vi "Dashboard Main.vi"() -> ()   [LabVIEW 2017]
uses:
  <vilib>/Rock Robotics/WPI/DriverStation/WPI_DriverStationAllianceInfo.ctl
  <vilib>/Utility/miscctls.llb/LVRowAndColumnTypeDef.ctl
  <vilib>/event_ctls.llb/eventvkey.ctl
  <vilib>/Rock Robotics/Network Tables/NT Read Numeric Array.vi
  <vilib>/Rock Robotics/WPI/Dashboard/WPI_DashboardLogging Global.vi
  <vilib>/Rock Robotics/Network Tables/NT Write Numeric Array.vi
  <vilib>/Rock Robotics/Network Tables/NT Write Boolean.vi
  <vilib>/Rock Robotics/Network Tables/NT Read Boolean.vi
panel:
  out "NT Connection":bool=TRUE
  in  "Camera Settings Right":T1={"Frame Rate"=15, "Compression"=30, "Size"=1, "DB Camera Config"=FALSE} {"Frame Rate" scale=1.0..30.0; "Compression" scale=100.0..-1.0; "Size" items=["640x480", "320x240", "160x120"]}
  in  "Camera Name Right":string(combo)="No Camera Selection"
  out "Camera Info":cluster{"Mbps LED":bool, "Mbps":dbl, "fps":dbl}={"Mbps LED"=FALSE, "Mbps"=0.17652911574406902, "fps"=9.930486593843098} {"fps" format="%#.1g"; "Mbps" format="%#.1g"}
  in  "Camera Settings":T1={"Frame Rate"=10, "Compression"=66, "Size"=2, "DB Camera Config"=FALSE} {"Frame Rate" scale=1.0..30.0; "Compression" scale=100.0..-1.0; "Size" items=["640x480", "320x240", "160x120"]}
  in  "TCP":refnum<k5>
  in  "Rec Mode":enum32{"Stop", "Record", "Playback"}(radio)
  out "Robot IP":string="10.17.12.2"
  out "Image Message":string="Timeout in Camera Communications"
  in  "Dashboard Tab":T2(tab)
  in  "Reset":bool
  out "HasCube":bool
  out "Mode":T3(ring)
  out "Gyro":dbl(knob)=-172.57 scale=-180.0..180.0
  out "Elevator":dbl(slide)=5.727272727272727 scale=-10.0..80.0
  out "LeftEncoder":dbl=817.74403425
  out "RightEncoder":dbl=362.091195
  out "Bottom":bool
  out "Top":bool
  out "Camera Image Right":T4(plugin-control)
  in  "DB/String 9":string
  in  "DB/String 8":string
  in  "DB/String 7":string
  in  "DB/String 6":string
  in  "DB/String 5":string
  in  "DB/String 4":string
  in  "DB/String 3":string
  in  "DB/String 2":string
  in  "DB/String 1":string
  in  "DB/String 0":string
  in  "DB/Slider 0":dbl(slide) scale=0.0..5.0
  in  "DB/Slider 1":dbl(slide) scale=0.0..5.0
  in  "DB/Slider 2":dbl(slide) scale=0.0..5.0
  in  "DB/Slider 3":dbl(slide) scale=0.0..5.0
  out "DB/LED 3":bool
  out "DB/LED 2":bool
  out "DB/LED 1":bool
  out "DB/LED 0":bool
  in  "DB/Button 3":bool
  in  "DB/Button 2":bool
  in  "DB/Button 1":bool
  in  "DB/Button 0":bool caption="New Name"
  in  "RR Delay":dbl
  in  "LR Delay":dbl
  in  "LL Delay":dbl
  in  "RRAction2":dbl
  in  "LRAction2":dbl
  in  "LLAction2":dbl
  in  "RRAction1":dbl
  in  "LRAction1":dbl
  in  "LLAction1":dbl
  in  "NotPurePursuit":bool
  in  "Battery Number":string
  out "?":bool=TRUE
  out "Opponent Right Switch":bool
  out "Center Left Scale":bool=TRUE
  out "Center Right Scale":bool
  out "Our Left Team Switch":bool=TRUE
  out "Our Right Team Switch":bool
  in  "Position":u32=3
  in  "RLAction1":dbl
  in  "RLAction2":dbl
  in  "RL Delay":dbl
  in  "Test Slider":dbl(slide) scale=0.0..100.0 scale format="%#_3g"
  in  "On/Off":bool caption="Solenoid"
  in  "Test Name":u16(ring) items=["Select the test to run..."]
  in  "Test Tree":string(tree)
  in  "Motor":cluster{"Value":dbl, "Enable":bool} {"Value" scale=-1.0..1.0 scale format="%#_3g"}
  out "Progress":T5 {"Test Progress" scale=0.0..100.0}
  in  "Rev/Fwd":cluster{"Forward":bool, "Reverse":bool}
  in  "Test Ring":u16(ring) items=["Monochrome", "Color"]
  out "Cmd Status":string
  in  "Execute Command":bool
  in  "Command Params":string[][](table)
  in  "Command Selection":i32(listbox)
  in  "CheckList":i32(listbox)
  out "Tree":string(tree)
  out "Camera Image":T4(plugin-control)
  in  "Camera Name":string(combo)="Camera"
  # "Don't use this row"
  # "HW"
  # "HW"
  # "Switch/Scale Positions"
  # "1Cube"
  # "2Cube"
  # "Delay"
  # "Left"
  # "Left"
  # "Right"
  # "Left"
  # "Left"
  # "Right"
  # "Right"
  # "Right"
  # "Action Key:\n0 = Do Nothing\n1 = Go Switch\n2 = Go Scale"
  # "1"
  # "2"
  # "3"
  # "4"
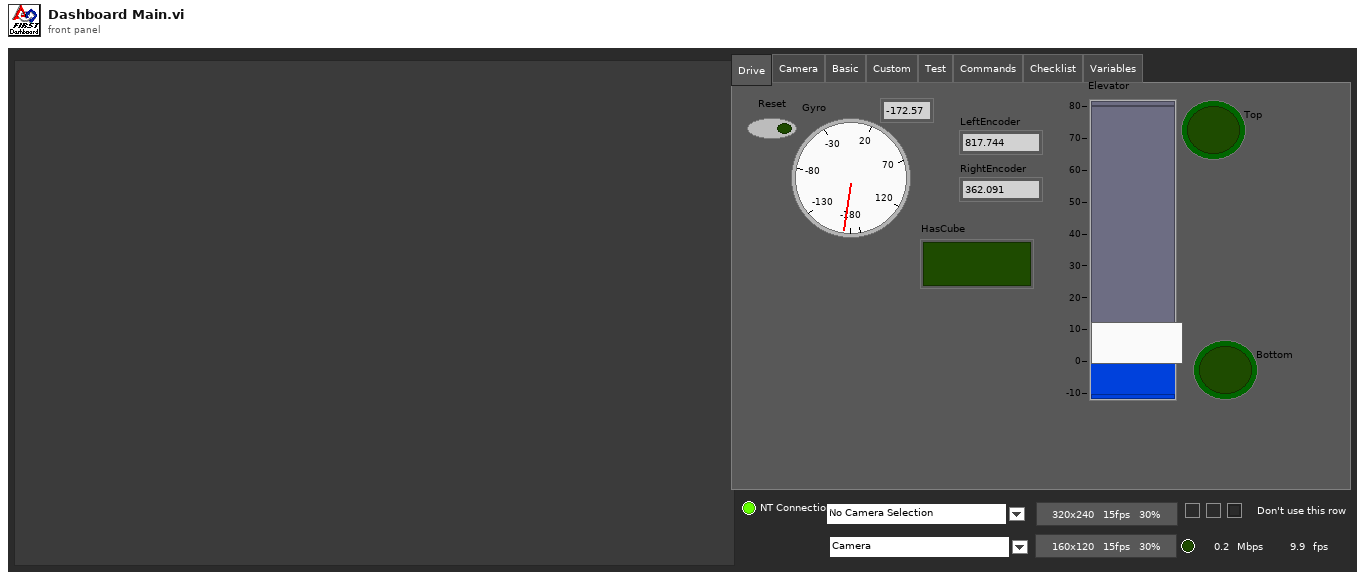
[diagram p1: front panel]
types:
  T1 = cluster{"Frame Rate":i32, "Compression":i32, "Size":u16, "DB Camera Config":bool}
  T2 = enum32{"Drive", "Camera", "Basic", "Custom", "Test", "Commands", "Checklist", "Variables"}
  T3 = enum8{"Tele-Op Disabled", "Tele-Op Enabled", "Auto Disabled", "Auto Enabled", "Test Disabled", "Test Enabled", "Disconnected", "No Code", "E-Stop"}
  T4 = typedef "IMAQ Image.ctl" = refnum<image>
  T5 = cluster{"Test Progress":u8, "Test Progress Text":string}
  T6 = cluster{"Save Path":path, "Interval (s)":dbl, "Keep":i32}
  T7 = typedef "Image Type" = u32
  T8 = cluster{"IDs":cluster{"RPC field ID":u16, "Unique ID":u16}, "String":string}
  T9 = cluster{"Camera Image":refnum<vi>, "Dashboard Tab":refnum<vi>, "Rec Mode":refnum<vi>, "Test Slider":refnum<vi>, "On/Off ":refnum<vi>, "Test Ring":refnum<vi>, "Rev/Fwd":refnum<vi>, "Test Name":refnum<vi>, "Motor":refnum<vi>, "Progress":refnum<vi>, "CheckList":refnum<vi>, "Tree":refnum<vi>, "Test Tree":refnum<vi>, "Command Params":refnum<vi>, "Command Selection":refnum<vi>, "Execute Command":refnum<vi>, "Cmd Status":refnum<vi>, "Camera Settings":refnum<vi>, "Camera Name":refnum<vi>, "Camera Info":refnum<vi>, "Camera Settings Right":refnum<vi>, "Camera Name Right":refnum<vi>, "Camera Image Right":refnum<vi>}
  T10 = cluster{"Error Strings":string, "Disable Counts":cluster{u16, u16}, "Rail Faults":cluster{u16, u16, u16}, "Robot IP":string, "DB Mode":u8, "Event Info":cluster{"Name":string, "Type":u8, "Number":u16, "Replay":u8}}
  T11 = cluster{"Storage":cluster{"Disk Free":u64, "RAM Block":u32, "RAM free":u32}, "CPU Utilization":cluster{"CPU % ISR":sgl, "CPU % Time Crit":sgl, "CPU % Timed Str":sgl, "CPU % High":sgl, "CPU % Above":sgl, "CPU % Normal":sgl, "CPU % Low":sgl}, "CAN":cluster{"% Bus Utilization":sgl, "Bus Off Cnt":u32, "TX_FIFO Full Cnt":u32, "Receive Error Cnt":u8, "Transmit Error Cnt":u8}, "HID":cluster{"HID Outputs":u32, "Rumble Low":u16, "Rumble High":u16}[]}
  T12 = cluster{"Status bits":cluster{"Test Mode":bool, "Autonomous":bool, "Enabled":bool, "Code Start":bool, "Brownout":bool, "Reserved 2":bool, "Reserved 3":bool, "E-Stop":bool}, "Code Trace":cluster{"Disabled":bool, "TeleOp":bool, "Auto":bool, "Test":bool}, "Controller Type":enum16{"unknown", "cRIO", "roboRio"}, "Code?":enum16{"unknown", "noCode", "code"}, "Battery V":dbl}
  T13 = cluster{"Control Bits":cluster{"TestMode":bool, "Autonomous":bool, "Enabled":bool, "FMS Present":bool, bool, bool, bool, "E-Stop":bool}, "Team Station ":u8, "Countdown":sgl, "Joystick Values":cluster{"Axes":dbl[], "Buttons":bool[], "POVs":i16[]}[]}
  T14 = cluster{"Axes":dbl[], "Buttons":bool[], "POVs":i16[]}[]
  T15 = cluster{"Axes":dbl[], "Buttons":bool[], "POVs":i16[]}
  T16 = cluster{"Camera Name":string, string, "Saved DB Images Info":cluster{"Save Path":path, "Interval (s)":dbl, "Keep":i32}}
  T17 = cluster{"Camera Name Right":string, string, "Saved DB Images Info":cluster{"Save Path":path, "Interval (s)":dbl, "Keep":i32}}
  T18 = cluster{"Operation":enum16{"Update", "Clear"}, "Color Box":u32}[]
  T19 = typedef "eventvkey.ctl" = enum16{"ASCII", "Enter", "Return", "Shift", "Ctrl", "Alt", "Cmd", "Opt", "Caps", "NumLock", "Clear", "Break", "Up", "Down", "Left", "Right", "Insert", "Delete", "Home", "End", "PageUp", "PageDown", "Escape", "Help", "Pause", "ScrollLock", "F1", "F2", "F3", "F4", "F5", "F6", "F7", "F8", "F9", "F10", "F11", "F12", "F13", "F14", "F15", "F16", "F17", "F18", "F19", "F20", "F21", "F22", "F23", "F24", "Play", "VolumeUp", "VolumeDown", "Mute", "Two Byte Char"}
  T20 = cluster{"Image Size":bool, "Image Type":bool, "Pixel Value":bool, "ROI Information":bool, "Zoom Factor":bool}
  T21 = cluster{"Operation":enum16{"Update", "Clear"}, "Color Box":u32}
  T22 = typedef "LVRowAndColumnTypeDef.ctl" = cluster{"Row":i32, "Column":i32}
  T23 = cluster{"Shift":bool, "Ctrl":bool, "Alt":bool, "Cmd":bool, "Opt":bool}
  T24 = typedef "WPI_DriverStationAllianceInfo.ctl" = enum16{"Red", "Blue", "Invalid"}
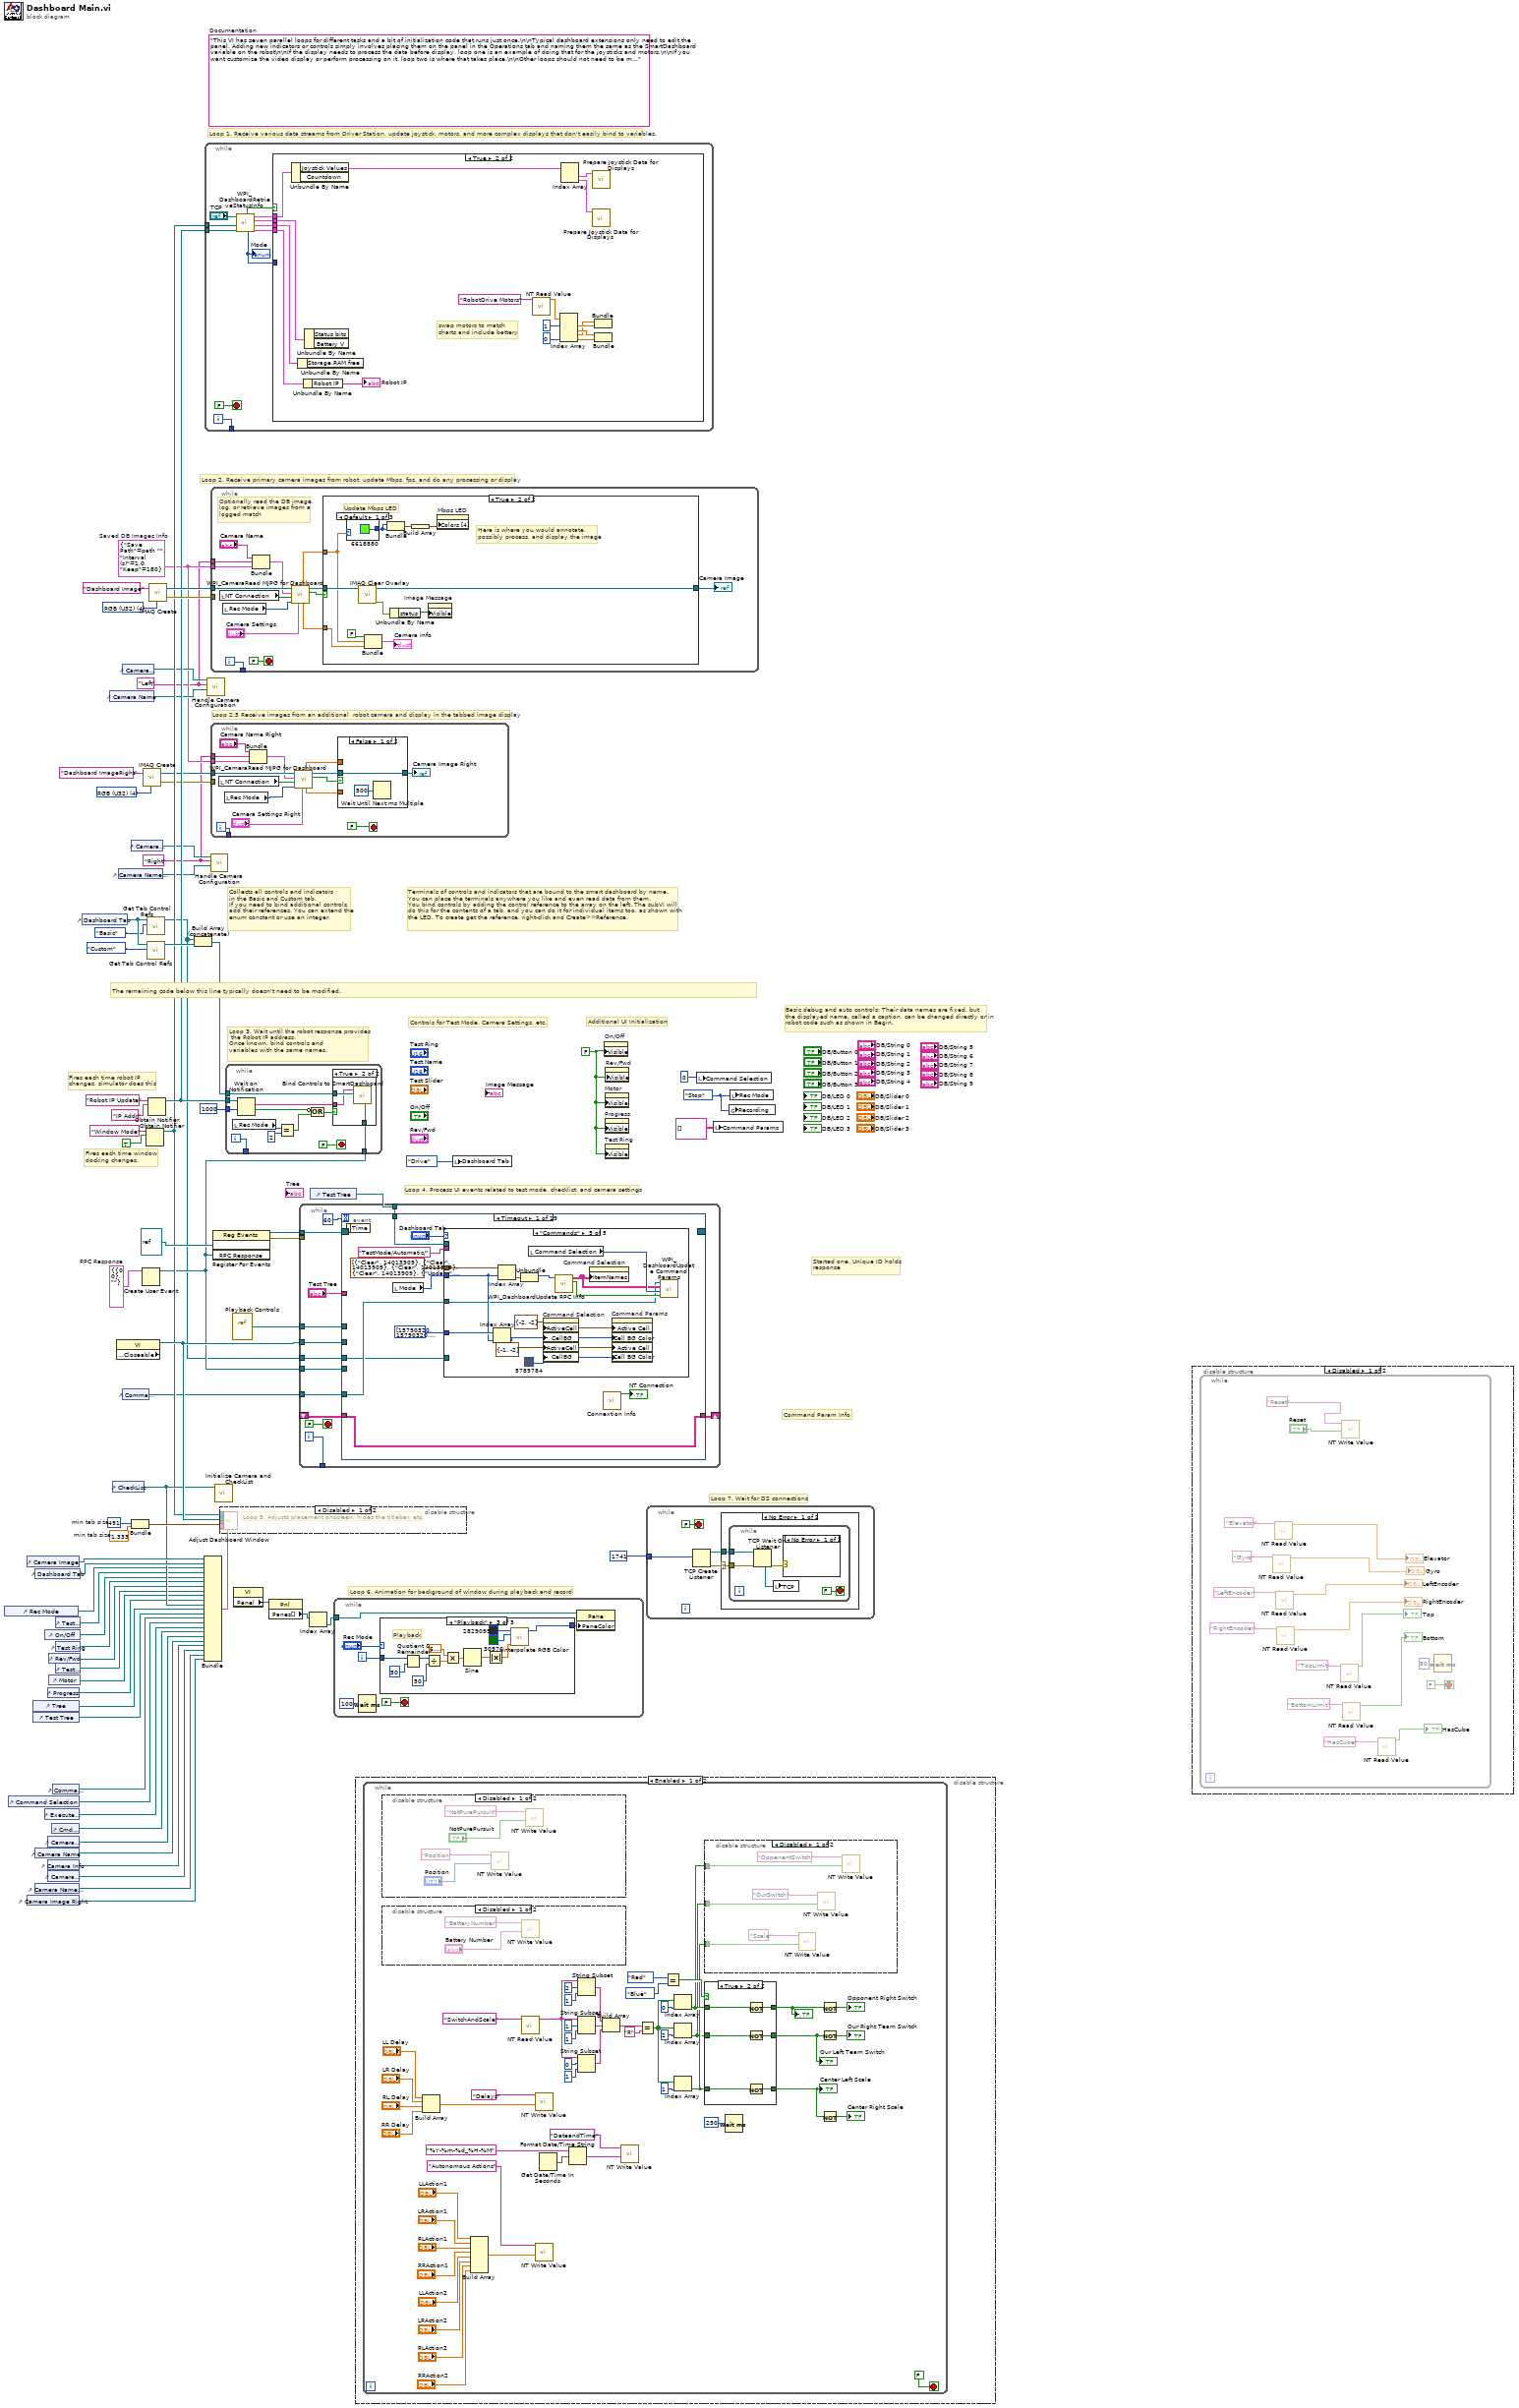
[diagram p0: block diagram]
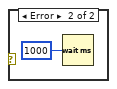
[diagram p10: hidden frame]
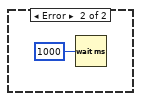
[diagram p11: hidden frame]
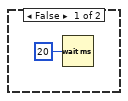
[diagram p12: hidden frame]
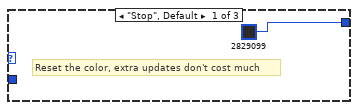
[diagram p13: hidden frame]
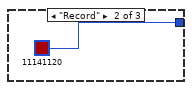
[diagram p14: hidden frame]
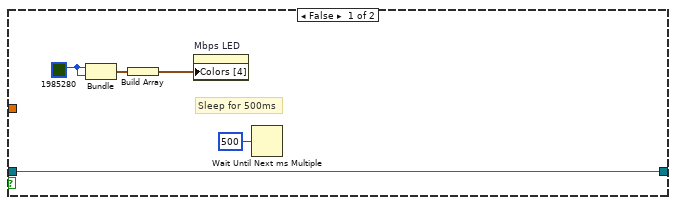
[diagram p16: hidden frame]
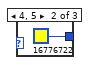
[diagram p17: hidden frame]
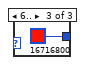
[diagram p18: hidden frame]
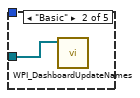
[diagram p20: hidden frame]
diagram:
  w4 = T6 {"Save Path"=path "", "Interval (s)"=1.0, "Keep"=180}  # Saved DB Images Info
  w3 = "Right"
  w2 = "Left"
  w14 = T7 4 items=["Grayscale (U8)", "Grayscale (I16)", "Grayscale (SGL)", "Complex (CSG)", "RGB (U32)", "HSL (U32)", "RGB (U64)"] ("Image Type")
  w28 = T8 {"IDs"={"RPC field ID"=0, "Unique ID"=0}, "String"=""}  # RPC Response
  w49 = 491  # min tab size
  w48 = 1.333  # min tab size
  w56 = enum32{"Stop", "Record", "Playback"}."Stop" ("Rec Mode")
  w34 = FALSE ("Visible")
  (unwired) "This VI has seven parallel loops for different tasks and a bit of initialization code that runs just once.\n\nTypical dashboard extensions only need to edit the panel. Adding new indicators or controls simply involves placing them on the panel in the Operations tab and naming them the same as the SmartDashboard variable on the robot\n\nIf the display needs to process the data before display, loop one is an example of doing that for the joysticks and motors.\n\nIf you want customize the video display or perform processing on it, loop two is where that takes place.\n\nOther loops should not need to be modified. They are pretty standard, and document the task they perform."  # Documentation
  w73 = T7 4 items=["Grayscale (U8)", "Grayscale (I16)", "Grayscale (SGL)", "Complex (CSG)", "RGB (U32)", "HSL (U32)", "RGB (U64)"] ("Image Type")
  # "Loop 2.5 Receive images from an additional  robot camera and display in the tabbed image display"
  # "Command Param Info"
  # "Started one, Unique ID holds\nresponse"
  # "Loop 7. Wait for DS connections"
  # "Basic debug and auto controls: Their data names are fixed, but\nthe displayed name, called a caption, can be changed directly or in\nrobot code such as shown in Begin."
  # "Controls for Test Mode, Camera Settings, etc."
  # "Additional UI Initialization"
  # "Loop 6. Animation for background of window during playback and record"
  # "Fires each time robot IP\nchanges, simulator does this"
  # "Fires each time window\ndocking changes."
  # "Collects all controls and indicators\nin the Basic and Custom tab.\nIf you need to bind additional controls,\nadd their references. You can extend the\nenum constant or use an integer."
  # "The remaining code below this line typically doesn't need to be modified."
  # "Loop 4. Process UI events related to test mode, checklist, and camera settings"
  # "Terminals of controls and indicators that are bound to the smart dashboard by name.\nYou can place the terminals anywhere you like and even read data from them.\nYou bind controls by adding the control reference to the array on the left. The subVI will\ndo this for the contents of a tab, and you can do it for individual items too, as shown with\nthe LED. To create get the reference, right-click and Create>>Reference."
  # "Loop 3. Wait until the robot response provides\n the Robot IP address.\nOnce known, bind controls and\nvariables with the same names."
  # "Loop 1. Receive various data streams from Driver Station, update joystick, motors, and more complex displays that don't easily bind to variables."
  # "Loop 2. Receive primary camera images from robot, update Mbps, fps, and do any processing or display"
  n1 = control-ref of="Rec Mode"() -> (w40:refnum<vi>)
  n2 = control-ref of="Command Selection"() -> (w27:refnum<vi>)
  n3 = control-ref of="Camera Image Right"() -> (w7:refnum<vi>)
  n4 = control-ref of="Camera Image"() -> (w51:refnum<vi>)
  n5 = control-ref of="Tree"() -> (w44:refnum<vi>)
  n6 = control-ref of="Test Tree"() -> (w43:refnum<vi>)
  n7 = control-ref of="Dashboard Tab"() -> (w50:refnum<vi>)
  n8 = control-ref of="Camera Name"() -> (w18:refnum<vi>)
  n9 = control-ref of="Camera Name Right"() -> (w8:refnum<vi>)
  n10 = control-ref of="Execute Command"() -> (w29:refnum<vi>)
  n11 = control-ref of="On/Off"() -> (w38:refnum<vi>)
  n12 = control-ref of="Progress"() -> (w35:refnum<vi>)
  n13 = control-ref of="Camera Settings"() -> (w19:refnum<vi>)
  n14 = control-ref of="Camera Info"() -> (w17:refnum<vi>)
  n15 = control-ref of="Camera Settings Right"() -> (w9:refnum<vi>)
  n16 = control-ref of="Rev/Fwd"() -> (w36:refnum<vi>)
  n17 = control-ref of="Motor"() -> (w41:refnum<vi>)
  n18 = control-ref of="Cmd Status"() -> (w23:refnum<vi>)
  n19 = control-ref of="Command Params"() -> (w30:refnum<vi>)
  n20 = control-ref of="Test Slider"() -> (w39:refnum<vi>)
  n21 = control-ref of="Test Ring"() -> (w37:refnum<vi>)
  n22 = control-ref of="Test Name"() -> (w42:refnum<vi>)
  n23 = control-ref of="Dashboard Tab"() -> (w54:refnum<vi>)
  n24 = control-ref of="Camera Name"() -> (w20:refnum<vi>)
  n25 = control-ref of="CheckList"() -> (w45:refnum<vi>)
  n26 = property class="VI" props=["Front Panel.Closeable"]() -> (reference out=w55:refnum<vi>)  [unwired: 2 in, 2 out]
  n27 = control-ref of="Camera Name Right"() -> (w10:refnum<vi>)
  n28 = control-ref of="Camera Settings"() -> (w21:refnum<vi>)
  n29 = control-ref of="Command Params"() -> (w22:refnum<vi>)
  n30 = control-ref of="Camera Settings Right"() -> (w11:refnum<vi>)
  n31 = Bundle("min tab size"=w49, "min tab size"=w48) -> (w47:cluster{"min tab size":i32, "min tab size":dbl})  [unwired: 1 in]
  n32 = Create User Event(user event datatype=w28) -> (user event=w24:refnum<user-event>)  [unwired: 1 in, 1 out]
  n33 = call "IMAQ Create"("Image Name"="Dashboard ImageRight", "Image Type"=w14) -> ("New Image"=w13:T4, "error out"=w12:errorcluster)  [unwired: 2 in, 1 out]
  n34 = Obtain Notifier(name (unnamed)="Window Mode", notification data type=TRUE) -> (notifier out=w32:refnum<notifier>)  [unwired: 2 in, 2 out]
  n35 = call <vilib>:"Get Tab Control Refs.vi"("Page Index"=T2."Basic" ("Dashboard Tab"), "TabControl in"=w54) -> ("ControlsOnPage"=w16:refnum<vi>[])  [unwired: 9 in]
  n36 = call <vilib>:"Get Tab Control Refs.vi"("Page Index"=T2."Custom" ("Dashboard Tab"), "TabControl in"=w54) -> ("ControlsOnPage"=w53:refnum<vi>[])  [unwired: 9 in]
  n37 = Obtain Notifier(name (unnamed)="Robot IP Update", notification data type="IP Addr" ("name (unnamed)")) -> (notifier out=w33:refnum<notifier>)  [unwired: 2 in, 2 out]
  n38 = call "IMAQ Create"("Image Name"="Dashboard Image", "Image Type"=w73) -> ("New Image"=w71:T4, "error out"=w70:errorcluster)  [unwired: 2 in, 1 out]
  n39 = Build Array (concatenate)(w16, w53) -> (w52:refnum<vi>[])
  n40 = Bundle("Camera Image"=w51, "Dashboard Tab"=w50, "Rec Mode"=w40, "Test Slider"=w39, "On/Off"=w38, "Test Ring"=w37, "Rev/Fwd"=w36, "Test Name"=w42, "Motor"=w41, "Progress"=w35, "CheckList"=w45, "Tree"=w44, "Test Tree"=w43, "Command Params"=w30, "Command Selection"=w27, "Execute Command"=w29, "Cmd Status"=w23, "Camera Settings"=w19, "Camera Name"=w18, "Camera Info"=w17, "Camera Settings Right"=w9, "Camera Name Right"=w8, "Camera Image Right"=w7) -> (w46:T9)  [unwired: 1 in]
  n41 = while {
    tunnel: [w83] -> _
    tunnel: w33 -> [w77]
    tunnel: w32 -> [w74]
    i -> [w83]
    stop <- FALSE stop-if-true
    n42 = call <vilib>:"WPI_DashboardRetrieveStatusInfo.vi"("Binding Refnum"=w77, "Window Mode Notifier"=w74, "TCP Cnx"="TCP") -> ("Power and Errors"=w78:T10, "Robot Metrics"=w81:T11, "Status Info"=w82:T12, "Control Info"=w79:T13, "Robot Mode"=w76:T3, "Process?"=w80:bool)  [unwired: 3 in]
    "Mode" <- w76
    n43 = case shown="True" w80 {
      tunnel: w82 -> [_ w101]
      tunnel: w81 -> [_ w100]
      tunnel: w79 -> [_ w99]
      tunnel: w78 -> [_ w98]
      tunnel: w76 -> [_ _]
      frame False {
        n44 = Wait (ms)(milliseconds to wait=u32 20) -> ()  [unwired: 1 out]
      }
      frame True {
        # "swap motors to match\ncharts and include battery"
        n45 = Unbundle By Name(w99) -> ("Joystick Values"=w91:T14)  [unwired: 1 out]
        n46 = Unbundle By Name(w100) -> ()  [unwired: 1 out]
        n47 = Unbundle By Name(w98) -> ("Robot IP"=→"Robot IP":string)
        n48 = Unbundle By Name(w101) -> ()  [unwired: 2 out]
        n49 = call-poly <vilib>:"NT Read Value.vi"("Name"="RobotDrive Motors") -> ("Numeric Array"=w87:dbl[])  [unwired: 9 in, 1 out]
        n50 = Index Array(array=w87, index #1=1, index #4=0) -> (element #1=w93:dbl, element #2=w94:dbl, element #3=w92:dbl, element #4=w97:dbl)  [unwired: 2 in]
        n51 = Index Array(array=w91) -> (element #1=w90:T15, element #2=w89:T15)  [unwired: 2 in]
        n52 = call "Prepare Joystick Data for Displays.vi"("Joystick Values"=w89) -> ()  [unwired: 8 in, 3 out]
        n53 = call "Prepare Joystick Data for Displays.vi"("Joystick Values"=w90) -> ()  [unwired: 8 in, 3 out]
        n54 = Bundle("Numeric"=w92, "Numeric"=w93) -> ()  [unwired: 1 in, 1 out]
        n55 = Bundle("Numeric"=w94, "Numeric"=w97) -> ()  [unwired: 1 in, 1 out]
      }
    }
  }
  n56 = call "Handle Camera Configuration.vi"("CameraNameRef"=w20, "Display Name"=w2, "ClusterRef"=w21) -> ()  [unwired: 9 in]
  n57 = while {
    tunnel: w71 -> [w114]
    tunnel: w70 -> [_]
    tunnel: [w115] -> _
    tunnel: w4 -> [w105]
    tunnel: w2 -> [w102]
    i -> [w115]
    stop <- FALSE stop-if-true
    # "Optionally read the DB image,\nlog, or retrieve images from a\nlogged match"
    n58 = local read "NT Connection"() -> (w106:bool)
    n59 = local read "Rec Mode"() -> (w110:enum32{"Stop", "Record", "Playback"})
    n60 = Bundle("Camera Name"="Camera Name", w102, "Saved DB Images Info"=w105) -> (w104:T16)  [unwired: 1 in]
    n61 = call <vilib>:"WPI_CameraRead MJPG for Dashboard.vi"("Camera Settings"="Camera Settings", "Rec Mode"=w110, "NT Connection"=w106, "Capture Info"=w104, "Refnum in"=w114) -> ("Active"=w112:bool, "Refnum out"=w113:T4, "FPS"=w111:dbl, "Bandwidth (Mbps)"=w109:dbl)  [unwired: 3 in]
    n62 = case shown="True" w112 {
      tunnel: w113 -> [w117 w128]
      tunnel: w109 -> [_ w125]
      tunnel: w111 -> [_ w126]
      tunnel: [w117 w122] -> w107
      frame False {
        w119 = u32 1985280 ("Color Box")
        # "Sleep for 500ms"
        n63 = Bundle("Color Box"=w119, "Color Box"=w119) -> (w120:cluster{"Color Box":u32, "Color Box":u32})  [unwired: 1 out]
        n64 = Build Array(w120) -> (w118:cluster{"Color Box":u32, "Color Box":u32}[])
        n65 = property on="Mbps LED" class="Bool (strict)"("Colors [4]"=w118) -> ()  [unwired: 2 in, 2 out]
        n66 = Wait Until Next ms Multiple(millisecond multiple=u32 500) -> ()  [unwired: 1 out]
      }
      frame True {
        # "Here is where you would annotate,\npossibly process, and display the image"
        # "Update Mbps LED"
        n67 = case shown="Default" w125 {
          tunnel: [u32 6618880 ("Color Box") u32 16776722 ("Color Box") u32 16716800 ("Color Box")] -> w129
          frame Default {
          }
          frame 4, 5 {
          }
          frame 6.. {
          }
        }
        n68 = call "IMAQ Clear Overlay"("Image"=w128) -> ("error out"=w131:errorcluster, "Image Out"=w122:T4)  [unwired: 2 in, 7 out]
        n69 = Bundle(FALSE, "Bandwidth (Mbps)"=w125, "FPS"=w126) -> (→"Camera Info":cluster{bool, "Bandwidth (Mbps)":dbl, "FPS":dbl})  [unwired: 1 in]
        n70 = Bundle("Color Box"=w129, "Color Box"=w129) -> (w130:cluster{"Color Box":u32, "Color Box":u32})  [unwired: 1 out]
        n71 = Unbundle By Name(w131) -> ("status"=w132:bool)
        n72 = Build Array(w130) -> (w127:cluster{"Color Box":u32, "Color Box":u32}[])
        n73 = property on="Image Message" class="Str"("Visible"=w132) -> ()  [unwired: 2 in, 2 out]
        n74 = property on="Mbps LED" class="Bool (strict)"("Colors [4]"=w127) -> ()  [unwired: 2 in, 2 out]
      }
    }
    "Camera Image" <- w107
  }
  n75 = while {
    tunnel: w13 -> [w150]
    tunnel: w12 -> [_]
    tunnel: [w145] -> _
    tunnel: w4 -> [w139]
    tunnel: w3 -> [w136]
    i -> [w145]
    stop <- FALSE stop-if-true
    n76 = local read "NT Connection"() -> (w140:bool)
    n77 = local read "Rec Mode"() -> (w149:enum32{"Stop", "Record", "Playback"})
    n78 = Bundle("Camera Name Right"="Camera Name Right", w136, "Saved DB Images Info"=w139) -> (w138:T17)  [unwired: 1 in]
    n79 = call <vilib>:"WPI_CameraRead MJPG for Dashboard.vi"("Camera Settings"="Camera Settings Right", "Rec Mode"=w149, "NT Connection"=w140, "Capture Info"=w138, "Refnum in"=w150) -> ("Active"=w144:bool, "Refnum out"=w147:T4, "FPS"=w142:dbl, "Bandwidth (Mbps)"=w143:dbl)  [unwired: 3 in]
    n80 = case shown="False" w144 {
      tunnel: w147 -> [w151 w153]
      tunnel: w143 -> [_ _]
      tunnel: w142 -> [_ _]
      tunnel: [w151 w153] -> w141
      frame False {
        n81 = Wait Until Next ms Multiple(millisecond multiple=u32 500) -> ()  [unwired: 1 out]
      }
      frame True {
      }
    }
    "Camera Image Right" <- w141
  }
  n82 = call "Handle Camera Configuration.vi"("CameraNameRef"=w10, "Display Name"=w3, "ClusterRef"=w11) -> ()  [unwired: 9 in]
  n83 = register-events(refnum<vi> refnum, w24) -> (reference out=w60:refnum<event-registration>, error out=w59:errorcluster)  [unwired: 2 in]
  n84 = call "Initialize Camera and CheckList.vi"("ListBox in"=w45) -> ()  [unwired: 11 in]
  n85 = disable-structure shown="Disabled" {
    disable-tunnel: w55 -> [w157 _]
    disable-tunnel: w47 -> [w156 _]
    disable-tunnel: w46 -> [w155 _]
    disable-tunnel: w32 -> [w154 _]
    frame Disabled {
      # "Loop 5. Adjusts placement onscreen, hides the titlebar, etc."
      n86 = call "Adjust Dashboard Window.vi"("Sizing Refnums"=w155, "Size Constraints"=w156, "VI"=w157, "WIn Mode"=w154) -> ()  [unwired: 8 in]
    }
    frame Enabled {
    }
  }
  n87 = while {
    tunnel: w52 -> [w169]
    tunnel: w33 -> [w167]
    tunnel: [w165] -> _
    tunnel: u32 1000 ("milliseconds to wait") -> [w164]
    tunnel: w24 -> [w158]
    i -> [w165]
    stop <- FALSE stop-if-true
    n88 = local read "Rec Mode"() -> (w160:enum32{"Stop", "Record", "Playback"})
    n89 = Wait on Notification(notifier=w167, timeout in ms (-1)=w164) -> (notification=w166:string, timed out?=w162:bool)  [unwired: 2 in, 2 out]
    n90 = Equal?(x=w160, y=u16 2 ("Rec Mode")) -> (x = y?=w161:bool)
    n91 = Compound Arithmetic op=OR(invert w162, w161) -> (w163:bool)
    n92 = case shown="True" w163 {
      tunnel: w169 -> [_ w172]
      tunnel: w166 -> [_ w171]
      tunnel: w158 -> [_ w170]
      frame False {
      }
      frame True {
        n93 = call <vilib>:"Bind Controls to SmartDashboard.vi"("RPC ref"=w170, "Bound Control Refs"=w172, "Server IP Address"=w171) -> ()  [unwired: 9 in]
      }
    }
  }
  n94 = vi-ref "Playback Controls.vi"() -> (w61:refnum<vi>)
  n95 = property class="VI"() -> ("Panel"=w63:refnum<vi>)  [unwired: 2 in, 2 out]
  n96 = property class="Pnl"(reference=w63) -> ("Panes[]"=w64:refnum<vi>[])  [unwired: 1 in, 2 out]
  n97 = Index Array(array=w64) -> (element=w62:refnum<vi>)  [unwired: 1 in]
  n98 = control-ref of="Test Tree"() -> (w65:refnum<vi>)
  n99 = while {
    tunnel: [w182] -> _
    tunnel: w65 -> [w181]
    tunnel: w61 -> [w180]
    tunnel: w60 -> [w179]
    tunnel: w59 -> [_]
    tunnel: w55 -> [w178]
    tunnel: w24 -> [w177]
    tunnel: w22 -> [w176]
    shift-right: [w175] -> _
    shift-left: _ -> [w174]
    tunnel: w16 -> [w173]
    i -> [w182]
    stop <- FALSE stop-if-true
    n100 = event shown="[0] Timeout" {
      selector: w179 -> [_ _ _ _ _ _ _ _ _ _ _ _ _ _ _ _ _ _ _]
      dyn-events: [_ _ _ _ _ _ _ _ _ _ _ _ _ _ w436 _ _ _ _] -> _
      timeout: u32 60 ("milliseconds to wait") -> [_ _ _ _ _ _ _ _ _ _ _ _ _ _ _ _ _ _ _]
      tunnel: w181 -> [w194 _ _ _ _ _ _ _ _ _ _ _ _ _ _ _ _ _ _]
      tunnel: "Test Tree" -> [_ _ _ _ _ _ _ _ _ w403 w411 w413 w417 w425 _ _ _ _ _]
      tunnel: w180 -> [_ _ _ _ _ _ _ _ _ _ _ _ _ _ w438 _ w456 _ _]
      tunnel: w178 -> [_ _ _ _ _ _ _ _ _ _ _ _ _ _ w434 _ _ _ _]
      tunnel: w177 -> [_ _ _ _ _ _ _ _ _ _ _ _ _ _ w432 _ _ _ _]
      tunnel: w176 -> [w189 _ _ _ w354 _ _ _ _ _ _ _ _ _ _ _ _ _ _]
      tunnel: [w188 w237 w339 w344 w352 w361 w371 w378 w390 w402 w409 w412 w416 w424 w431 w451 w453 w457 w470] -> w175
      tunnel: w174 -> [w188 w237 w339 w344 w352 _ _ w378 w390 w402 w409 w412 w416 w424 w431 w451 w453 w457 w470]
      tunnel: w173 -> [w186 _ _ _ _ _ _ _ _ _ _ _ _ _ _ _ _ _ _]
      event Timeout {
        n101 = event-data() -> ()  [unwired: 1 in, 1 out]
        n102 = local read "Mode"() -> (w191:T3)
        n103 = case shown="\"Commands\"" "Dashboard Tab" {
          tunnel: w194 -> [_ _ w210 _ _]
          tunnel: "TestMode/Automatic/" ("Name Pattern") -> [_ _ w209 _ _]
          tunnel: T18 [{"Operation"=enum."Clear", "Color Box"=14013909}, {"Operation"=enum."Clear", "Color Box"=14013909}, {"Operation"=enum."Clear", "Color Box"=14013909}, {"Operation"=enum."Clear", "Color Box"=14013909}, {"Operation"=enum."Update", "Color Box"=14013909}, {"Operation"=enum."Update", "Color Box"=16777215}, {"Operation"=enum."Clear", "Color Box"=14013909}, {"Operation"=enum."Clear", "Color Box"=14013909}, {"Operation"=enum."Clear", "Color Box"=14013909}] -> [_ _ w202 _ w230]
          tunnel: w191 -> [_ _ w201 _ w229]
          tunnel: u32[] [15790320, 15790320, 15790320, 15790320, 16777215, 16777215, 15790320, 15790320, 15790320] -> [_ _ _ _ w235]
          tunnel: w189 -> [_ _ _ _ w223]
          tunnel: w186 -> [_ w196 _ _ _]
          frame "Custom", Default {
          }
          frame "Basic" {
            n104 = call <vilib>:"WPI_DashboardUpdateNames.vi"("Controls on Tab"=w196) -> ()  [unwired: 11 in]
          }
          frame "Test" {
            w208 = -2 ("Active Item:Row Number")
            n105 = Index Array(array=w202, index=w201) -> (element=w203:T21)
            n106 = Unbundle(w203) -> ("Operation"=w204:enum16{"Update", "Clear"}, "Color Box"=w205:u32)
            n107 = call <vilib>:"NT Read String.vi"("Name"="TestMode/TestName") -> ("String"=w199:string)  [unwired: 9 in, 1 out]
            n108 = call <vilib>:"NT Read and Format Entries as Tree.vi"("Operation"=w204, "Name Pattern"=w209, "Tree Refnum"=w210) -> ()  [unwired: 7 in, 2 out]
            n109 = case shown="\"\"" w199 {
              tunnel: "TestMode/TestProgress" ("Name") -> [w212 _]
              tunnel: "TestMode/TestProgressText" ("Name") -> [w211 _]
              frame Default {
                n110 = call <vilib>:"NT Read Number.vi"("Name"=w212) -> ("Numeric"=w213:dbl)  [unwired: 9 in, 1 out]
                n111 = call <vilib>:"NT Read String.vi"("Name"=w211) -> ("String"=w214:string)  [unwired: 9 in, 1 out]
                n112 = Bundle("Numeric"=w213, "String"=w214) -> (→"Progress":cluster{"Numeric":dbl, "String":string})  [unwired: 1 in]
              }
              frame "" {
                n113 = property on="Progress" class="Clust (strict)"("Visible"=FALSE) -> ()  [unwired: 2 in, 2 out]
                n114 = local write "Test Name"(u16 0) -> ()
              }
            }
            n115 = property on="Test Tree" class="Tree (strict)"("Active Item Row Number"=w208, "ActiveColNum"=w208, "CellBG"=w205, "Active Item Row Number"=-1 ("Active Item:Row Number"), "CellBG"=u32 5789784 ("Color Box")) -> ()  [unwired: 2 in, 2 out]
          }
          frame "Variables" {
            w220 = string[] ["CameraPublisher", "Usage", "DB"]  # Items to initially close
            n116 = First Call?() -> (First Call?: T/F=w221:bool)
            n117 = control-ref of="Tree"() -> (w222:refnum<vi>)
            n118 = Select(t=w220, s=w221, f=string[] []) -> (s? t:f=w218:string[])
            n119 = call <vilib>:"NT Read and Format Entries as Tree.vi"("Tags to  Close"=w218, "Tree Refnum"=w222) -> ()  [unwired: 8 in, 2 out]
          }
          frame "Commands" {
            w231 = u32 5789784 ("Color Box")
            w232 = T22 {"Row"=-1, "Column"=-2} ("Active Cell:Active Cell")
            w234 = T22 {"Row"=-2, "Column"=-2} ("Active Cell:Active Cell")
            n120 = Index Array(array=w235, index=w229) -> (element=w233:u32)
            n121 = Index Array(array=w230, index=w229) -> (element=w228:T21)
            n122 = Unbundle(w228) -> ("Operation"=w227:enum16{"Update", "Clear"})  [unwired: 1 out]
            n123 = local read "Command Selection"() -> (w226:i32)
            n124 = property on="Command Selection" class="MCListbox (strict)"("ActiveCell"=w234, "CellBG"=w233, "ActiveCell"=w232, "CellBG"=w231) -> ()  [unwired: 2 in, 2 out]
            n125 = call <vilib>:"WPI_DashboardUpdate RPC Info.vi"("Operation"=w227) -> ("update"=w225:bool, "commands"=w224:string[][])  [unwired: 9 in]
            n126 = property on="Command Selection" class="MCListbox (strict)"("ItemNames"=w224) -> ()  [unwired: 2 in, 2 out]
            n127 = property on="Command Params" class="Tbl (strict)"("Active Cell"=w234, "Cell BG Color"=w233, "Active Cell"=w232, "Cell BG Color"=w231) -> ()  [unwired: 2 in, 2 out]
            n128 = call <vilib>:"WPI_DashboardUpdate Command Params.vi"("Update"=w225, "NewVal"=w226, "Commands"=w224, "Param Tbl"=w223) -> ()  [unwired: 7 in, 1 out]
          }
        }
        n129 = call <vilib>:"Connextion Info.vi"() -> ("Connected"=→"NT Connection":bool)  [unwired: 10 in, 1 out]
      }
      event "Test Tree": Value Change {
        # "Show appropriate\ncontrols"
        n130 = event-data() -> ("CtlRef"=w240:refnum<vi>, "NewVal"=w238:string)  [unwired: 1 in]
        n131 = call <vilib>:"WPI_UtilitiesGetTreeIOName.vi"("NewVal"=w238, "TreeControl in"=w240) -> ("I/O Name"=w241:string)  [unwired: 9 in]
        n132 = case shown="\"Camera\"" w241 {
          selector: w241 -> [_ w248 _ w270 w279 _]
          tunnel: w238 -> [_ _ w267 w269 _ w286]
          tunnel: cluster{string[]}[] [{["640x480", "320x240", "160x120"]}, {["Auto", "Fixed indoor", "Fixed outdoor 1", "Fixed outdoor 2", "Fixed fluorescent 1", "Fixed fluorescent 2", "Hold current"]}, {["Auto", "Flicker-free 50 Hz", "Flicker-free 60 Hz", "Hold current"]}, {["None", "Prioritize frame rate", "Prioritize image quality"]}, {["Monochrome", "Color"]}] -> [_ _ _ _ _ w285]
          frame Default {
            w243 = FALSE ("Visible")
            w242 = FALSE ("Visible")
            n133 = property on="Motor" class="Clust (strict)"("Visible"=w242) -> ()  [unwired: 2 in, 2 out]
            n134 = property on="Test Ring" class="Ring (strict)"("Visible"=w242) -> ()  [unwired: 2 in, 2 out]
            n135 = property on="Rev/Fwd" class="Clust (strict)"("Visible"=w243) -> ()  [unwired: 2 in, 2 out]
            n136 = property on="On/Off" class="Bool (strict)"("Visible"=w243) -> ()  [unwired: 2 in, 2 out]
            n137 = property on="Test Slider" class="Slide (strict)"("Visible"=w243) -> ()  [unwired: 2 in, 2 out]
          }
          frame "Analog Out", "Motor", "PWM" {
            w249 = FALSE ("Visible")
            n138 = case shown="\"Analog Out\"" w248 {
              tunnel: [1.0 ("Value") -1.0 ("Value") 0.0 ("Value")] -> w247
              tunnel: [255.0 ("Value") 1.0 ("Value") 5.0 ("Value")] -> w246
              tunnel: [128.0 ("Value") 0.0 ("Value") 0.0 ("Value")] -> w245
              tunnel: [64.0 ("Value") 0.5 ("Value") 1.0 ("Value")] -> w244
              frame "PWM" {
              }
              frame "Motor", Default {
              }
              frame "Analog Out" {
              }
            }
            n139 = property on="Motor" class="Clust (strict)"("Visible"=TRUE) -> ()  [unwired: 2 in, 2 out]
            n140 = property on="Value" class="Slide (strict)"("Value"=w245, "Scale.Minimum"=w247, "Scale.Maximum"=w246, "Scale.Increment"=w244) -> ()  [unwired: 2 in, 2 out]
            n141 = property on="On/Off" class="Bool (strict)"("Visible"=w249) -> ()  [unwired: 2 in, 2 out]
            n142 = property on="Test Slider" class="Slide (strict)"("Visible"=w249) -> ()  [unwired: 2 in, 2 out]
            n143 = property on="Test Ring" class="Ring (strict)"("Visible"=w249) -> ()  [unwired: 2 in, 2 out]
            n144 = property on="Rev/Fwd" class="Clust (strict)"("Visible"=w249) -> ()  [unwired: 2 in, 2 out]
          }
          frame "Servo" {
            w265 = FALSE ("Visible")
            n145 = call <vilib>:"NT Read Number.vi"("Name"=w267) -> ("Numeric"=w266:dbl)  [unwired: 9 in, 1 out]
            n146 = property on="Test Slider" class="Slide (strict)"("Visible"=TRUE, "Scale.Maximum"=170.0 ("Scale.Range:Maximum")) -> ()  [unwired: 2 in, 2 out]
            n147 = local write "Test Slider"(w266) -> ()
            n148 = property on="Motor" class="Clust (strict)"("Visible"=w265) -> ()  [unwired: 2 in, 2 out]
            n149 = property on="Rev/Fwd" class="Clust (strict)"("Visible"=w265) -> ()  [unwired: 2 in, 2 out]
            n150 = property on="On/Off" class="Bool (strict)"("Visible"=w265) -> ()  [unwired: 2 in, 2 out]
            n151 = property on="Test Ring" class="Ring (strict)"("Visible"=w265) -> ()  [unwired: 2 in, 2 out]
          }
          frame "Relay", "Solenoid" {
            w268 = FALSE ("Visible")
            n152 = property on="Motor" class="Clust (strict)"("Visible"=w268) -> ()  [unwired: 2 in, 2 out]
            n153 = property on="Test Slider" class="Slide (strict)"("Visible"=w268) -> ()  [unwired: 2 in, 2 out]
            n154 = Search and Replace String(input string=w269, search string="/Value  **", replace string="/Direction") -> (result string=w275:string)  [unwired: 5 in, 3 out]
            n155 = property on="Test Ring" class="Ring (strict)"("Visible"=w268) -> ()  [unwired: 2 in, 2 out]
            n156 = call <vilib>:"NT Read String.vi"("Name"=w275) -> ("String"=w273:string)  [unwired: 9 in, 1 out]
            n157 = Equal?(x="Both directions", y=w273) -> (x = y?=w271:bool)
            n158 = Not(x=w271) -> (.not. x?=w272:bool)
            n159 = property on="Rev/Fwd" class="Clust (strict)"("Visible"=w271) -> ()  [unwired: 2 in, 2 out]
            n160 = property on="On/Off" class="Bool (strict)"("Visible"=w272, "Caption.Text"=w270) -> ()  [unwired: 2 in, 2 out]
          }
          frame "Compressor", "Digital Out" {
            w278 = FALSE ("Visible")
            # "Get direction and finish"
            n161 = property on="Motor" class="Clust (strict)"("Visible"=w278) -> ()  [unwired: 2 in, 2 out]
            n162 = property on="Test Slider" class="Slide (strict)"("Visible"=w278) -> ()  [unwired: 2 in, 2 out]
            n163 = property on="Test Ring" class="Ring (strict)"("Visible"=w278) -> ()  [unwired: 2 in, 2 out]
            n164 = property on="On/Off" class="Bool (strict)"("Visible"=TRUE, "Caption.Text"=w279) -> ()  [unwired: 2 in, 2 out]
            n165 = property on="Rev/Fwd" class="Clust (strict)"("Visible"=FALSE) -> ()  [unwired: 2 in, 2 out]
          }
          frame "Camera" {
            n166 = call <vilib>:"Get Last Path Segment.vi"("String in"=w286) -> ("String out"=w287:string)  [unwired: 10 in]
            n167 = property on="On/Off" class="Bool (strict)"("Visible"=FALSE) -> ()  [unwired: 2 in, 2 out]
            n168 = property on="Motor" class="Clust (strict)"("Visible"=FALSE) -> ()  [unwired: 2 in, 2 out]
            n169 = property on="Rev/Fwd" class="Clust (strict)"("Visible"=FALSE) -> ()  [unwired: 2 in, 2 out]
            n170 = case shown="\"White Balance  **\"" w287 {
              tunnel: w286 -> [w293 w302 w311 w320 w329 _ w335]
              tunnel: w285 -> [w291 w299 w308 w317 w326 _ _]
              frame "Size  **" {
                n171 = Index Array(array=w291) -> (element=w290:cluster{string[]})  [unwired: 1 in]
                n172 = call <vilib>:"NT Read String.vi"("Name"=w293) -> ("String"=w292:string)  [unwired: 9 in, 1 out]
                n173 = Unbundle(w290) -> (w288:string[])
                n174 = Match First String(2:w288, 3:w292) -> (0:w289:i32)  [unwired: 1 out]
                n175 = property on="Test Ring" class="Ring (strict)"("Value"=w289, "Strings []"=w288) -> ()  [unwired: 2 in, 2 out]
                n176 = property on="Test Ring" class="Ring (strict)"("Visible"=TRUE) -> ()  [unwired: 2 in, 2 out]
                n177 = property on="Test Slider" class="Slide (strict)"("Visible"=FALSE) -> ()  [unwired: 2 in, 2 out]
              }
              frame "White Balance  **" {
                n178 = Index Array(array=w299, index=1) -> (element=w300:cluster{string[]})
                n179 = call <vilib>:"NT Read String.vi"("Name"=w302) -> ("String"=w301:string)  [unwired: 9 in, 1 out]
                n180 = Unbundle(w300) -> (w297:string[])
                n181 = Match First String(2:w297, 3:w301) -> (0:w296:i32)  [unwired: 1 out]
                n182 = property on="Test Ring" class="Ring (strict)"("Value"=w296, "Strings []"=w297) -> ()  [unwired: 2 in, 2 out]
                n183 = property on="Test Ring" class="Ring (strict)"("Visible"=TRUE) -> ()  [unwired: 2 in, 2 out]
                n184 = property on="Test Slider" class="Slide (strict)"("Visible"=FALSE) -> ()  [unwired: 2 in, 2 out]
              }
              frame "Exposure  **" {
                n185 = Index Array(array=w308, index=2) -> (element=w309:cluster{string[]})
                n186 = call <vilib>:"NT Read String.vi"("Name"=w311) -> ("String"=w310:string)  [unwired: 9 in, 1 out]
                n187 = Unbundle(w309) -> (w305:string[])
                n188 = Match First String(2:w305, 3:w310) -> (0:w306:i32)  [unwired: 1 out]
                n189 = property on="Test Ring" class="Ring (strict)"("Value"=w306, "Strings []"=w305) -> ()  [unwired: 2 in, 2 out]
                n190 = property on="Test Ring" class="Ring (strict)"("Visible"=TRUE) -> ()  [unwired: 2 in, 2 out]
                n191 = property on="Test Slider" class="Slide (strict)"("Visible"=FALSE) -> ()  [unwired: 2 in, 2 out]
              }
              frame "Exposure Priority  **" {
                n192 = Index Array(array=w317, index=3) -> (element=w318:cluster{string[]})
                n193 = call <vilib>:"NT Read String.vi"("Name"=w320) -> ("String"=w319:string)  [unwired: 9 in, 1 out]
                n194 = Unbundle(w318) -> (w314:string[])
                n195 = Match First String(2:w314, 3:w319) -> (0:w315:i32)  [unwired: 1 out]
                n196 = property on="Test Ring" class="Ring (strict)"("Value"=w315, "Strings []"=w314) -> ()  [unwired: 2 in, 2 out]
                n197 = property on="Test Ring" class="Ring (strict)"("Visible"=TRUE) -> ()  [unwired: 2 in, 2 out]
                n198 = property on="Test Slider" class="Slide (strict)"("Visible"=FALSE) -> ()  [unwired: 2 in, 2 out]
              }
              frame "Color Enable  **" {
                n199 = Index Array(array=w326, index=4) -> (element=w327:cluster{string[]})
                n200 = call <vilib>:"NT Read String.vi"("Name"=w329) -> ("String"=w328:string)  [unwired: 9 in, 1 out]
                n201 = Unbundle(w327) -> (w323:string[])
                n202 = Match First String(2:w323, 3:w328) -> (0:w324:i32)  [unwired: 1 out]
                n203 = property on="Test Ring" class="Ring (strict)"("Value"=w324, "Strings []"=w323) -> ()  [unwired: 2 in, 2 out]
                n204 = property on="Test Ring" class="Ring (strict)"("Visible"=TRUE) -> ()  [unwired: 2 in, 2 out]
                n205 = property on="Test Slider" class="Slide (strict)"("Visible"=FALSE) -> ()  [unwired: 2 in, 2 out]
              }
              frame Default {
                n206 = property on="Test Ring" class="Ring (strict)"("Visible"=FALSE) -> ()  [unwired: 2 in, 2 out]
                n207 = property on="Test Slider" class="Slide (strict)"("Visible"=FALSE) -> ()  [unwired: 2 in, 2 out]
              }
              frame "Brightness  **", "Color Level  **", "Compression  **", "FPS  **", "Sharpness  **" {
                n208 = call <vilib>:"NT Read Number.vi"("Name"=w335) -> ("Numeric"=w334:dbl)  [unwired: 9 in, 1 out]
                n209 = local write "Test Slider"(w334) -> ()
                n210 = property on="Test Slider" class="Slide (strict)"("Visible"=TRUE, "Scale.Maximum"=100.0 ("Scale.Range:Maximum")) -> ()  [unwired: 2 in, 2 out]
                n211 = property on="Test Ring" class="Ring (strict)"("Visible"=FALSE) -> ()  [unwired: 2 in, 2 out]
              }
            }
          }
        }
        n212 = property on="Progress" class="Clust (strict)"("Visible"=FALSE) -> ()  [unwired: 2 in, 2 out]
      }
      event "Test Name": Mouse Enter {
        # "Populate the ring with the list of tests"
        n213 = event-data() -> ()  [unwired: 1 in, 1 out]
        n214 = call <vilib>:"NT Read String Array.vi"("Name"="TestMode/TestList") -> ("String Array"=w343:string[])  [unwired: 9 in, 1 out]
        n215 = Build Array (concatenate)("Select the test to run...", w343) -> (w342:string[])
        n216 = property on="Test Name" class="Ring (strict)"("Strings []"=w342) -> ()  [unwired: 2 in, 2 out]
      }
      event "Test Name": Value Change {
        w345 = FALSE ("Visible")
        # "Tell the robot the test name to run"
        n217 = event-data() -> ("NewVal"=w349:u16)  [unwired: 1 in]
        n218 = property on="Test Name" class="Ring (strict)"() -> ("Strings []"=w350:string[])  [unwired: 2 in, 2 out]
        n219 = local write "Progress"(T5 {"Test Progress"=0, "Test Progress Text"=""} ("Progress")) -> ()
        n220 = Index Array(array=w350, index=w349) -> (element=w348:string)
        n221 = call <vilib>:"NT Write String.vi"("String"=w348, "Name"="TestMode/TestName") -> ()  [unwired: 9 in, 1 out]
        n222 = property on="Progress" class="Clust (strict)"("Visible"=TRUE) -> ()  [unwired: 2 in, 2 out]
        n223 = property on="Motor" class="Clust (strict)"("Visible"=w345) -> ()  [unwired: 2 in, 2 out]
        n224 = property on="Test Slider" class="Slide (strict)"("Visible"=w345) -> ()  [unwired: 2 in, 2 out]
        n225 = property on="On/Off" class="Bool (strict)"("Visible"=w345) -> ()  [unwired: 2 in, 2 out]
        n226 = property on="Rev/Fwd" class="Clust (strict)"("Visible"=w345) -> ()  [unwired: 2 in, 2 out]
        n227 = property on="Test Ring" class="Ring (strict)"("Visible"=w345) -> ()  [unwired: 2 in, 2 out]
      }
      event "Command Selection": Value Change {
        # "Get the params and show in table"
        n228 = event-data() -> ("NewVal"=w355:i32)  [unwired: 1 in]
        n229 = property on="Command Selection" class="MCListbox (strict)"() -> ("ItemNames"=w353:string[][])  [unwired: 2 in, 2 out]
        n230 = call <vilib>:"WPI_DashboardUpdate Command Params.vi"("NewVal"=w355, "Commands"=w353, "Param Tbl"=w354) -> ()  [unwired: 8 in, 1 out]
      }
      event "Execute Command": Value Change {
        # "Started one, Unique ID holds\nresponse"
        n231 = event-data() -> ()  [unwired: 1 in, 1 out]
        n232 = property on="Command Selection" class="MCListbox (strict)"() -> ("ItemNames"=w366:string[][])  [unwired: 2 in, 2 out]
        n233 = Index Array(array=w366, index (row)="Command Selection", index (col)=0) -> (element=w364:string)
        n234 = call <vilib>:"Invoke Commands.vi"("Command Params"="Command Params", "Function Name"=w364) -> ("Params"=w360:u8, "Started"=w359:bool)  [unwired: 7 in, 1 out]
        n235 = Array Subset(array="Command Params", length (row)=w360) -> (w361:string[][])  [unwired: 3 in]
        n236 = Select(t="Executing" ("Cmd Status"), s=w359, f="" ("Cmd Status")) -> (s? t:f=→"Cmd Status":string)
      }
      event "Command Selection": Double Click {
        n237 = event-data() -> ("Row"=w374:i32)  [unwired: 1 in]
        n238 = property on="Command Selection" class="MCListbox (strict)"() -> ("ItemNames"=w377:string[][])  [unwired: 2 in, 2 out]
        n239 = local read "Command Params"() -> (w373:string[][])
        n240 = Index Array(array=w377, index (row)=w374, index (col)=0) -> (element=w375:string)
        n241 = call <vilib>:"Invoke Commands.vi"("Command Params"=w373, "Function Name"=w375) -> ("Params"=w372:u8, "Started"=w367:bool)  [unwired: 7 in, 1 out]
        n242 = Array Subset(array=w373, length (row)=w372) -> (w371:string[][])  [unwired: 3 in]
        n243 = Select(t="Executing" ("Cmd Status"), s=w367, f="" ("Cmd Status")) -> (s? t:f=w368:string)
        n244 = local write "Cmd Status"(w368) -> ()
      }
      event "CheckList": Double Click {
        # "Shift clears all"
        # "Update symbols on the listbox"
        n245 = event-data() -> ("PlatMods.Shift"=w379:bool, "Row"=w381:i32)  [unwired: 1 in]
        n246 = case shown="True" w379 {
          tunnel: w381 -> [w385 _]
          tunnel: 1 -> [w384 _]
          frame False {
            n247 = property on="CheckList" class="LstBox (strict)"() -> ("Item Symbols"=w383:i32[])  [unwired: 2 in, 2 out]
            n248 = Replace Array Subset(array=w383, new element=w384, index=w385) -> (w382:i32[])
            n249 = property on="CheckList" class="LstBox (strict)"("Item Symbols"=w382) -> ()  [unwired: 2 in, 2 out]
          }
          frame True {
            w386 = 0 ("Top Row")
            n250 = property on="CheckList" class="LstBox (strict)"() -> ("Number of Rows"=w388:u32)  [unwired: 2 in, 2 out]
            n251 = Initialize Array(0, w388) -> (w387:i32[])
            n252 = property on="CheckList" class="LstBox (strict)"("Top Row"=w386, "Value"=w386, "Item Symbols"=w387) -> ()  [unwired: 2 in, 2 out]
          }
        }
      }
      event "CheckList": Key Down {
        # "Update symbols on the listbox\nLeft and right keys check and uncheck"
        n253 = event-data() -> ("VKey"=w392:T19)  [unwired: 1 in]
        n254 = case shown="\"Left\", \"Right\"" w392 {
          selector: w392 -> [w397 _]
          tunnel: eventvkey."Left" ("VKey") -> [w395 _]
          frame "Left", "Right" {
            n255 = Equal?(x=w395, y=w397) -> (x = y?=w396:bool)
            n256 = Select(t=0, s=w396, f=1) -> (s? t:f=w398:i32)
            n257 = property on="CheckList" class="LstBox (strict)"() -> ("Item Symbols"=w401:i32[])  [unwired: 2 in, 2 out]
            n258 = Replace Array Subset(array=w401, new element=w398, index="CheckList") -> (w400:i32[])
            n259 = property on="CheckList" class="LstBox (strict)"("Item Symbols"=w400) -> ()  [unwired: 2 in, 2 out]
          }
          frame Default {
          }
        }
      }
      event "Motor.Enable": Value Change {
        # "When the test mode otor enable helper is set, update that\ntree row item's value"
        n260 = event-data() -> ("NewVal"=w407:bool)  [unwired: 1 in]
        n261 = Unbundle("Motor") -> ("Value"=w406:dbl)  [unwired: 1 out]
        n262 = Select(t=w406, s=w407, f=0.0) -> (s? t:f=w404:dbl)
        n263 = call <vilib>:"NT Write Number.vi"("Numeric"=w404, "Name"=w403) -> ()  [unwired: 9 in, 1 out]
      }
      event "Test Slider": Value Change {
        # "When the test mode slider helper is set, update that\ntree row item's value"
        n264 = event-data() -> ("NewVal"=w410:dbl)  [unwired: 1 in]
        n265 = call <vilib>:"NT Write Number.vi"("Numeric"=w410, "Name"=w411) -> ()  [unwired: 9 in, 1 out]
      }
      event "On/Off": Value Change {
        # "When the test mode on/off helper value is set, update that\ntree row item's value"
        n266 = event-data() -> ("NewVal"=w415:bool)  [unwired: 1 in]
        n267 = Boolean To (0,1)(Boolean=w415) -> (0, 1=w414:i16)
        n268 = call <vilib>:"NT Write Number.vi"("Numeric"=w414, "Name"=w413) -> ()  [unwired: 9 in, 1 out]
      }
      event "Rev/Fwd": Value Change {
        # "When the test mode helper value for relays is set, update that\ntree row item's value"
        n269 = event-data() -> ("NewVal.Forward"=w423:bool, "NewVal.Reverse"=w422:bool)  [unwired: 1 in]
        n270 = Boolean To (0,1)(Boolean=w423) -> (0, 1=w419:i16)
        n271 = Boolean To (0,1)(Boolean=w422) -> (0, 1=w421:i16)
        n272 = Negate(x=w421) -> (-x=w420:i16)
        n273 = Add(x=w419, y=w420) -> (x+y=w418:i16)
        n274 = call <vilib>:"NT Write Number.vi"("Numeric"=w418, "Name"=w417) -> ()  [unwired: 9 in, 1 out]
      }
      event "Test Ring": Value Change {
        # "When a test mode helper value is selected from the ring,\nset the tree item's variable to the string value"
        n275 = event-data() -> ("NewVal"=w427:u16)  [unwired: 1 in]
        n276 = property on="Test Ring" class="Ring (strict)"() -> ("Strings []"=w428:string[])  [unwired: 2 in, 2 out]
        n277 = Index Array(array=w428, index=w427) -> (element=w426:string)
        n278 = call <vilib>:"NT Write String.vi"("String"=w426, "Name"=w425) -> ()  [unwired: 9 in, 1 out]
      }
      event "Rec Mode": Value Change {
        # "Update globals for recording mode and path to read log from.\nClear when logging and let NetworkTables set path for vision to\nuse."
        n279 = event-data() -> ("NewVal"=w439:enum32{"Stop", "Record", "Playback"})  [unwired: 1 in]
        n280 = global write "WPI_DashboardLogging Global.vi" "Logging Filename"(path "") -> ()
        n281 = global write "WPI_DashboardLogging Global.vi" "Recording"(w439) -> ()
        n282 = case shown="\"Playback\"" w439 {
          tunnel: w438 -> [_ w441 w450]
          tunnel: [_ _ w449] -> w436
          tunnel: [_ _ w448] -> _
          tunnel: w434 -> [_ _ w446]
          tunnel: cluster{i32, i32} {-250, 170} -> [_ _ w445]
          tunnel: [_ _ T20 {"Image Size"=TRUE, "Image Type"=TRUE, "Pixel Value"=TRUE, "ROI Information"=TRUE, "Zoom Factor"=FALSE} ("Image Information Shown:All Elements")] -> w429
          tunnel: [_ _ TRUE ("Zoom Factor")] -> w430
          tunnel: w432 -> [_ _ w442]
          frame Default {
          }
          frame "Stop", "Record" {
            # "Place Window too"
            n283 = invoke class="VI" method="FP.Close"(reference=w441) -> (reference out=w440:refnum<vi>)  [unwired: 2 in, 2 out]
            n284 = invoke class="VI" method="Abort VI"(reference=w440) -> ()  [unwired: 2 in, 3 out]
          }
          frame "Playback" {
            n285 = call "Open Playback Panel.vi"("Offset"=w445, "DB VI Ref"=w446, "Playback in"=w450) -> ("Playback out"=w447:refnum<vi>)  [unwired: 8 in]
            n286 = register-events(w447, w442) -> (reference out=w449:refnum<event-registration>, error out=w448:errorcluster)  [unwired: 2 in]
          }
        }
        n287 = property on="Camera Image Right" class="ImageControl"("Image Information Shown"=w429, "Image Information Visible"=w430) -> ()  [unwired: 2 in, 2 out]
        n288 = property on="Camera Image" class="ImageControl"("Image Information Shown"=w429, "Image Information Visible"=w430) -> ()  [unwired: 2 in, 2 out]
        n289 = call <vilib>:"WPI_DashboardNT Log FieldName Cache.vi"("Operation"=enum16{"Lookup/Add", "Index", "Clear"}."Clear") -> ()  [unwired: 8 in, 3 out]
      }
      event Panel Close {
        w452 = enum32{"Stop", "Record", "Playback"}."Stop" ("Rec Mode")
        # "Playback window has been closed, abort"
        n290 = event-data() -> ()  [unwired: 1 in, 4 out]
        n291 = local write "Rec Mode"(w452) -> ()
        n292 = global write "WPI_DashboardLogging Global.vi" "Recording"(w452) -> ()
      }
      event Panel Close {
        # "Abort playback window and ourself"
        n293 = event-data() -> ()  [unwired: 1 in, 4 out]
        n294 = invoke class="VI" method="FP.Close"(reference=w456) -> (reference out=w455:refnum<vi>)  [unwired: 2 in, 2 out]
        n295 = invoke class="VI" method="Abort VI"(reference=w455) -> (error out=w454:errorcluster)  [unwired: 2 in, 2 out]
        n296 = invoke class="VI" method="Abort VI"(error in=w454) -> ()  [unwired: 2 in, 3 out]
      }
      event User Event {
        n297 = event-data() -> ("IDs"=w463:cluster{"RPC field ID":u16, "Unique ID":u16}, "String"=w462:string)  [unwired: 1 in]
        n298 = Bundle("IDs"=w463, "String"=w462) -> (w461:T8)  [unwired: 1 in]
        n299 = call <vilib>:"Retrieve RPC Response.vi"("RPC Response"=w461) -> ("Output"=w459:string[][])  [unwired: 10 in]
        n300 = Build Array (concatenate)(w457, w459) -> (w458:string[][])
        n301 = local write "Command Params"(w458) -> ()
        n302 = local write "Cmd Status"("" ("Cmd Status")) -> ()
      }
      event "Tree": Double Click {
        n303 = event-data() -> ("PlatMods"=w469:T23, "Tag"=w466:string)  [unwired: 1 in]
        n304 = Unbundle(w469) -> ("Shift"=w468:bool)  [unwired: 4 out]
        n305 = String Subset(string=w466, length (rest)=1 ("length (rest)")) -> (substring=w465:string)  [unwired: 1 in]
        n306 = Not(x=w468) -> (.not. x?=w467:bool)
        n307 = case shown="\"/\"" w465 {
          tunnel: w466 -> [_ w472]
          tunnel: w467 -> [_ w471]
          frame Default {
          }
          frame "/" {
            n308 = call <vilib>:"NT Update Persistence.vi"("Persistence"=w471, "Name"=w472) -> ()  [unwired: 9 in, 1 out]
          }
        }
      }
    }
  }
  n309 = while {
    tunnel: w62 -> [w474]
    i -> [w477]
    stop <- FALSE stop-if-true
    n310 = Wait (ms)(milliseconds to wait=u32 100) -> ()  [unwired: 1 out]
    n311 = case shown="\"Playback\"" "Rec Mode" {
      tunnel: w477 -> [_ _ w492]
      tunnel: [u32 2829099 ("Base Color") u32 11141120 ("Target Color") w481] -> w473
      frame "Stop", Default {
        # "Reset the color, extra updates don't cost much"
      }
      frame "Record" {
      }
      frame "Playback" {
        # "Playback"
        n312 = Quotient & Remainder(x=w492, y=u32 50 ("milliseconds to wait")) -> (x-y*floor(x/y)=w488:u32)  [unwired: 1 out]
        n313 = Divide(x=w488, y=u32 50 ("milliseconds to wait")) -> (x/y=w485:dbl)
        n314 = Multiply(x=6.283185307179586, y=w485) -> (x*y=w490:dbl)
        n315 = Sine(x=w490) -> (sin(x)=w489:dbl)
        n316 = Absolute Value(x=w489) -> (abs(x)=w482:dbl)
        n317 = call "Interpolate RGB Color.vi"("Proportion"=w482, "Target Color"=u32 30976, "Base Color"=u32 2829099) -> ("Result Color"=w481:u32)  [unwired: 8 in]
      }
    }
    n318 = property class="Pane"(reference=w474, "PaneColor"=w473) -> ()  [unwired: 1 in, 2 out]
  }
  n319 = disable-structure shown="Enabled" {
    frame Enabled {
      n320 = while {
        stop <- FALSE stop-if-true
        n321 = disable-structure shown="Disabled" {
          frame Disabled {
            n322 = call-poly <vilib>:"NT Write Value.vi"("Numeric"="Position", "Name"="Position") -> ()  [unwired: 9 in, 1 out]
            n323 = call-poly <vilib>:"NT Write Value.vi"("Boolean"="NotPurePursuit", "Name"="NotPurePursuit") -> ()  [unwired: 9 in, 1 out]
          }
          frame Enabled {
          }
        }
        n324 = disable-structure shown="Disabled" {
          frame Disabled {
            n325 = call-poly <vilib>:"NT Write Value.vi"("String"="Battery Number", "Name"="BatteryNumber") -> ()  [unwired: 9 in, 1 out]
          }
          frame Enabled {
          }
        }
        n326 = Build Array("LL Delay", "LR Delay", "RL Delay", "RR Delay") -> (w499:dbl[])
        n327 = Build Array("LLAction1", "LRAction1", "RLAction1", "RRAction1", "LLAction2", "LRAction2", "RLAction2", "RRAction2") -> (w503:dbl[])
        n328 = call-poly <vilib>:"NT Read Value.vi"("Name"="SwitchAndScale") -> ("String"=w511:string)  [unwired: 9 in, 1 out]
        n329 = call-poly <vilib>:"NT Write Value.vi"("Numeric Array"=w499, "Name"="Delays") -> ()  [unwired: 9 in, 1 out]
        n330 = call-poly <vilib>:"NT Write Value.vi"("Numeric Array"=w503, "Name"="Autonomous Actions") -> ()  [unwired: 9 in, 1 out]
        n331 = Get Date/Time In Seconds() -> (seconds since 1Jan1904=w540:timestamp)
        n332 = Format Date/Time String(time format string (%c)="%Y-%m-%d_%H-%M", seconds (now)=w540) -> (date/time string=w539:string)  [unwired: 1 in]
        n333 = String Subset(string=w511, offset (0)=2, length (rest)=1 ("length (rest)")) -> (substring=w533:string)
        n334 = String Subset(string=w511, offset (0)=1, length (rest)=1 ("length (rest)")) -> (substring=w532:string)
        n335 = String Subset(string=w511, offset (0)=0, length (rest)=1 ("length (rest)")) -> (substring=w531:string)
        n336 = Build Array(w533, w532, w531) -> (w530:string[])
        n337 = call-poly <vilib>:"NT Write Value.vi"("String"=w539, "Name"="DateandTime") -> ()  [unwired: 9 in, 1 out]
        n338 = Equal?(x=w530, y="R") -> (x = y?=w525:bool[])
        n339 = Equal?(x=WPI_DriverStationAllianceInfo."Red" ("y"), y=WPI_DriverStationAllianceInfo."Blue") -> (x = y?=w521:bool)
        n340 = Index Array(array=w525, index=0) -> (element=w514:bool)
        n341 = Index Array(array=w525, index=2) -> (element=w512:bool)
        n342 = Index Array(array=w525, index=1) -> (element=w513:bool)
        n343 = disable-structure shown="Disabled" {
          disable-tunnel: w514 -> [w552 _]
          disable-tunnel: w513 -> [w551 _]
          disable-tunnel: w512 -> [w550 _]
          frame Disabled {
            n344 = call-poly <vilib>:"NT Write Value.vi"("Boolean"=w551, "Name"="Scale") -> ()  [unwired: 9 in, 1 out]
            n345 = call-poly <vilib>:"NT Write Value.vi"("Boolean"=w550, "Name"="OurSwitch") -> ()  [unwired: 9 in, 1 out]
            n346 = call-poly <vilib>:"NT Write Value.vi"("Boolean"=w552, "Name"="OppenentSwitch") -> ()  [unwired: 9 in, 1 out]
          }
          frame Enabled {
          }
        }
        n347 = case shown="True" w521 {
          tunnel: w512 -> [w556 w560]
          tunnel: [w556 w559] -> w516
          tunnel: w513 -> [w558 w562]
          tunnel: [w558 w561] -> w519
          tunnel: w514 -> [w557 w564]
          tunnel: [w557 w563] -> w517
          frame False {
          }
          frame True {
            n348 = Not(x=w564) -> (.not. x?=w563:bool)
            n349 = Not(x=w560) -> (.not. x?=w559:bool)
            n350 = Not(x=w562) -> (.not. x?=w561:bool)
          }
        }
        "?" <- w517
        "Center Left Scale" <- w519
        "Our Left Team Switch" <- w516
        n351 = Wait (ms)(milliseconds to wait=u32 250) -> ()  [unwired: 1 out]
        n352 = Not(x=w517) -> (.not. x?=→"Opponent Right Switch":bool)
        n353 = Not(x=w516) -> (.not. x?=→"Our Right Team Switch":bool)
        n354 = Not(x=w519) -> (.not. x?=→"Center Right Scale":bool)
      }
    }
    frame Disabled {
    }
  }
  n355 = local write "Dashboard Tab"(T2."Drive" ("Dashboard Tab")) -> ()
  n356 = property on="On/Off" class="Bool (strict)"("Visible"=w34) -> ()  [unwired: 2 in, 2 out]
  n357 = property on="Motor" class="Clust (strict)"("Visible"=w34) -> ()  [unwired: 2 in, 2 out]
  n358 = property on="Progress" class="Clust (strict)"("Visible"=w34) -> ()  [unwired: 2 in, 2 out]
  n359 = property on="Test Ring" class="Ring (strict)"("Visible"=w34) -> ()  [unwired: 2 in, 2 out]
  n360 = property on="Rev/Fwd" class="Clust (strict)"("Visible"=w34) -> ()  [unwired: 2 in, 2 out]
  n361 = while {
    tunnel: u16 1741 ("timeout ms (25000)") -> [w566]
    stop <- FALSE stop-if-true
    n362 = TCP Create Listener(10:w566) -> (0:w565:errorcluster, 3:w567:refnum<k5>)  [unwired: 4 in, 1 out]
    n363 = case shown="No Error" w565 {
      selector: w565 -> [w569 _]
      tunnel: w567 -> [w570 _]
      frame No Error {
        n364 = while {
          tunnel: w570 -> [w573]
          tunnel: w569 -> [w572]
          stop <- FALSE stop-if-true
          n365 = TCP Wait On Listener(8:w572, 11:w573) -> (0:w574:errorcluster, 4:w575:refnum<k5>)  [unwired: 2 in, 3 out]
          n366 = local write "TCP"(w575) -> ()
          n367 = case shown="No Error" w574 {
            frame No Error {
            }
            frame Error {
              n368 = Wait (ms)(milliseconds to wait=u32 1000) -> ()  [unwired: 1 out]
            }
          }
        }
      }
      frame Error {
        n369 = Wait (ms)(milliseconds to wait=u32 1000) -> ()  [unwired: 1 out]
      }
    }
  }
  n370 = local write "Command Selection"(u16 0 ("milliseconds to wait")) -> ()
  n371 = local write "Command Params"(string[][] [] ("Command Params")) -> ()
  n372 = global write "WPI_DashboardLogging Global.vi" "Recording"(w56) -> ()
  n373 = local write "Rec Mode"(w56) -> ()
  n374 = disable-structure shown="Disabled" {
    frame Disabled {
      n375 = while {
        stop <- FALSE stop-if-true
        n376 = call-poly <vilib>:"NT Read Value.vi"("Name"="Gyro") -> ("Numeric"=→"Gyro":dbl)  [unwired: 9 in, 1 out]
        n377 = call-poly <vilib>:"NT Read Value.vi"("Name"="Elevator") -> ("Numeric"=→"Elevator":dbl)  [unwired: 9 in, 1 out]
        n378 = call-poly <vilib>:"NT Read Value.vi"("Name"="LeftEncoder") -> ("Numeric"=→"LeftEncoder":dbl)  [unwired: 9 in, 1 out]
        n379 = call-poly <vilib>:"NT Read Value.vi"("Name"="RightEncoder") -> ("Numeric"=→"RightEncoder":dbl)  [unwired: 9 in, 1 out]
        n380 = call-poly <vilib>:"NT Read Value.vi"("Name"="TopLimit") -> ("Boolean"=→"Top":bool)  [unwired: 9 in, 1 out]
        n381 = call-poly <vilib>:"NT Write Value.vi"("Boolean"="Reset", "Name"="Reset") -> ()  [unwired: 9 in, 1 out]
        n382 = call-poly <vilib>:"NT Read Value.vi"("Name"="BottomLimit") -> ("Boolean"=→"Bottom":bool)  [unwired: 9 in, 1 out]
        n383 = call-poly <vilib>:"NT Read Value.vi"("Name"="HasCube") -> ("Boolean"=→"HasCube":bool)  [unwired: 9 in, 1 out]
        n384 = Wait (ms)(milliseconds to wait=u32 80) -> ()  [unwired: 1 out]
      }
    }
    frame Enabled {
    }
  }
